vi "Gage_Core.vi"(8 "error in":errorcluster, 9 "SignalBufferQueue in":refnum<queue>, 10 "DWFCtrlQueue in":refnum<queue>) -> (0 "error out":errorcluster)   [LabVIEW 2013, in "Gage.lvlib"]
uses:
  <instrlib>/GageLv_uic/Gage.lvlib
  <instrlib>/AnalogDiscSDKLv/VIs/DWF_CtrlQueue.ctl
  <instrlib>/AnalogDiscSDKLv/VIs/DWF_State.ctl
  <instrlib>/GageLv_uic/VI/Gage_Configs.ctl
  <instrlib>/GageLv_uic/VI/Gage_PrivateStats.ctl
  <instrlib>/GageLv_uic/VI/Gage_DAQStatus.ctl
  <instrlib>/AnalogDiscSDKLv/VIs/DWF_Signal.ctl
  <vilib>/Utility/error.llb/DialogType.ctl
  <instrlib>/GageLv_uic/VI/SetSecondaryDataVIRef_Typedef.ctl
  <vilib>/Utility/error.llb/Error Cluster From Error Code.vi
  <vilib>/ErrorRing/Error Ring.xnode
  <instrlib>/AnalogDiscSDKLv/AnalogDiscSDKLv.lvlib
  <userlib>/Utility/ErrorLog_lib.lvlib
panel:
  in  "StartAll":bool
  out "Core#":i32
  in  "Get_ConfigAll":bool
  out "LiveStat":T1
  in  "Gage_Config":T3={"Acquisition"={"Sample Rate"=100000000.0, "Mode"=0, "Start (0)"=8192.0, "Depth"=8192.0, "Segment Size"=100.0, "Trigger Delay"=0.0, "Trigger Timeout"=0.0, "Trigger Holdoff"=0.0, "Clock mode"=enum."Internal"}, "Channels"=[{"Coupling"=0, "Differential Input"=FALSE, "Direct-to-ADC"=FALSE, "Range"=2000, "Impedance"=50, "DC Offset"=0, "Filter"=0}], "Trigger"={"Slope"=0, "Level"=0, "Source"=0, "External Range"=2000, "External Coupling"=0, "External"=TRUE, "Disable"=FALSE, "External Impedance"=0}, "Mode(Gage)"=enum."Continuous"} {"Trigger"."External Impedance" items=["50 Ohm", "HiZ"]; "Trigger"."External Coupling" items=["DC", "AC"]; "Trigger"."External Range" min=2000 max=10000 step=8000; "Trigger"."Slope" items=["Rising", "Falling"]; "Trigger"."Level" min=-100 max=100; "Trigger"."Source" min=0 max=64 step=1; "Channels"."Impedance" min=50 max=1000000 step=999950; "Channels"."Coupling" items=["DC", "AC"]; "Acquisition"."Segment Size" min=256.0 step=128.0; "Acquisition"."Trigger Delay" min=0.0 step=128.0; "Acquisition"."Trigger Timeout" format="%.0p"; "Acquisition"."Trigger Holdoff" min=0.0 step=128.0; "Acquisition"."Depth" min=256.0 step=128.0; "Acquisition"."Mode" items=["Single", "Dual", "Quad", "Octal"]; "Acquisition"."Sample Rate" format="%.0p"}
  out "Graph":sgl[][](graph)
  in  "fConfig":bool
  in  "Reset":bool
  in  "CloseAll":bool
  in  "Close":bool
  in  "Enumerate":bool
  in  "Open":bool
  in  "Quit":bool
  in  "Start":bool
  in  "ConfigAll":bool
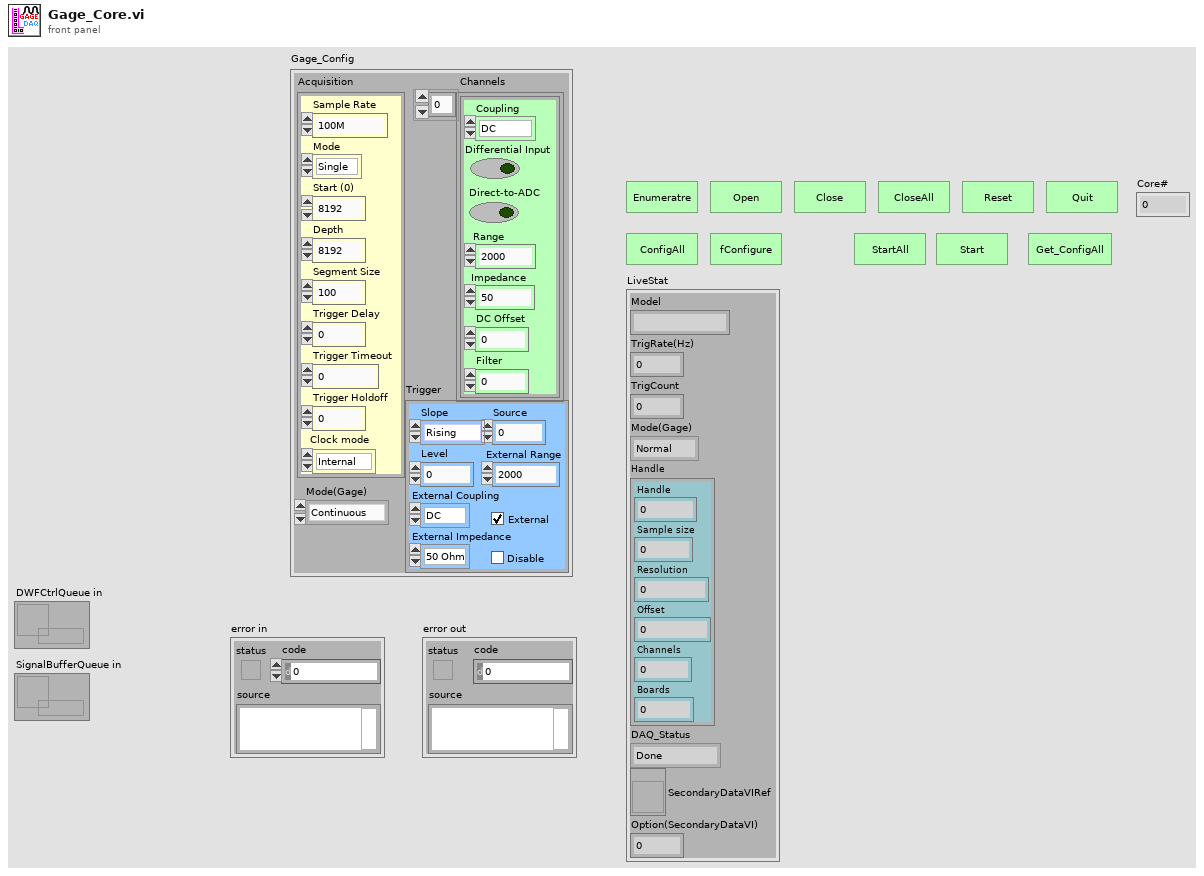
[diagram p1: front panel]
types:
  T1 = typedef "Gage.lvlib/Gage_PrivateStats.ctl" = cluster{"Model":string, "TrigRate(Hz)":dbl, "TrigCount":i32, "Mode(Gage)":enum16{"Normal", "Continuous", "MultiRecord", "HwAverage"}, "Handle":cluster{"Handle":u32, "Sample size":u32, "Resolution":i32, "Offset":i32, "Channels":u32, "Boards":u32}, "DAQ_Status":T2, "SecondaryDataVIRef":refnum<vi>, "Option(SecondaryDataVI)":i32}
  T2 = typedef "Gage.lvlib/Gage_DAQStatus.ctl" = enum16{"Done", "Armed", "Triggered", "Transfering"}
  T3 = typedef "Gage.lvlib/Gage_Configs.ctl" = cluster{"Acquisition":cluster{"Sample Rate":dbl, "Mode":u16, "Start (0)":dbl, "Depth":dbl, "Segment Size":dbl, "Trigger Delay":dbl, "Trigger Timeout":dbl, "Trigger Holdoff":dbl, "Clock mode":enum16{"Internal", "External", "Reference"}}, "Channels":cluster{"Coupling":u16, "Differential Input":bool, "Direct-to-ADC":bool, "Range":u32, "Impedance":u32, "DC Offset":i32, "Filter":i32}[], "Trigger":cluster{"Slope":u16, "Level":i32, "Source":i32, "External Range":u32, "External Coupling":u16, "External":bool, "Disable":bool, "External Impedance":u16}, "Mode(Gage)":enum16{"Normal", "Continuous", "MultiRecord", "HwAverage"}}
  T4 = typedef "DialogType.ctl" = u16
  T5 = typedef "AnalogDiscSDKLv.lvlib/DWF_Signal.ctl" = cluster{"tickcount":u32, "Signal":sgl[][], "SecondaryData":dbl[]}
  T6 = enum16{"Normal", "Continuous", "MultiRecord", "HwAverage"}
  T7 = typedef "AnalogDiscSDKLv.lvlib/DWF_CtrlQueue.ctl" = cluster{"DWF States":T8, "Variant":variant}
  T8 = typedef "AnalogDiscSDKLv.lvlib/DWF_State.ctl" = enum16{"Enumerate", "Open", "Close", "CloseAll", "Reset", "Quit", "==Settings==", "SetAcquisition_", "SetChannels_", "SetTrigger_", "SetAnalogTrigDetector_", "SetAll_AcquChTrig_", "fConfigurate", "fStart", "GetStatus", "_WaitForDone/Idle", "_GetData", "GetAcquisition", "GetChannels", "GetTrigger", "GetAll_AcquChTrig", "==Messaging==", "_PushDataOut", "GetStat_", "GetConfig_", "==ModeSetup==", "SetSignalBuffer_", "SetMode_", "SetSecondaryDataRef._", "==AnalogOut==", "GetChannelCount_AO", "fStart_AO", "SetChEnable_AO", "SetConfig_AO", "SetFuncData_AO", "SetOffset_AO_", "SetMasterNode_AO", "SetStates_AO", "SetSymetry_AO", "SetTriggerSource_AO", "==Trigger==", "ManualTrigger"}
  T9 = typedef "SetSecondaryDataVIRef_Typedef.ctl" = cluster{"SecondaryDataVIRef.":refnum<vi>, "Option":i32}
  T10 = cluster{"Handle":u32, "Sample size":u32, "Resolution":i32, "Offset":i32, "Channels":u32, "Boards":u32}
  T11 = cluster{"Sample Rate":dbl, "Mode":u16, "Start (0)":dbl, "Depth":dbl, "Segment Size":dbl, "Trigger Delay":dbl, "Trigger Timeout":dbl, "Trigger Holdoff":dbl, "Clock mode":enum16{"Internal", "External", "Reference"}}
  T12 = cluster{"Sample Rate":dbl, "Clock mode":enum16{"Internal", "External", "Reference"}, string, "Depth":dbl, "Segment Size":dbl, "Trigger Timeout":dbl, "Trigger Holdoff":dbl, "Trigger Delay":dbl}
  T13 = cluster{"Coupling":u16, "Differential Input":bool, "Direct-to-ADC":bool, "Range":u32, "Impedance":u32, "DC Offset":i32, "Filter":i32}[]
  T14 = cluster{string, "Differential Input":bool, "Direct-to-ADC":bool, "Range":u32, "Impedance":u32, "DC Offset":i32, "Filter":i32}
  T15 = cluster{"Slope":u16, "Level":i32, "Source":i32, "External Range":u32, "External Coupling":u16, "External":bool, "Disable":bool, "External Impedance":u16}
  T16 = cluster{string, "Level":i32, "Source":i32, "External Range":u32, string, "External":bool, "Disable":bool, string}
  T17 = cluster{string, "Level":i32, "Source":i32, "External Range":u32, string, "External":bool, "Disable":bool, string}[]
  T18 = cluster{"Handle":u32, "Sample Size":u32, "Resolution":i32, "Offset":i32, "Channels":u32, "Boards":u32}
  T19 = cluster{"Coupling":u16, "Differential Input":bool, "Direct-to-ADC":bool, "Range":u32, "Impedance":u32, "DC Offset":i32, "Filter":i32}
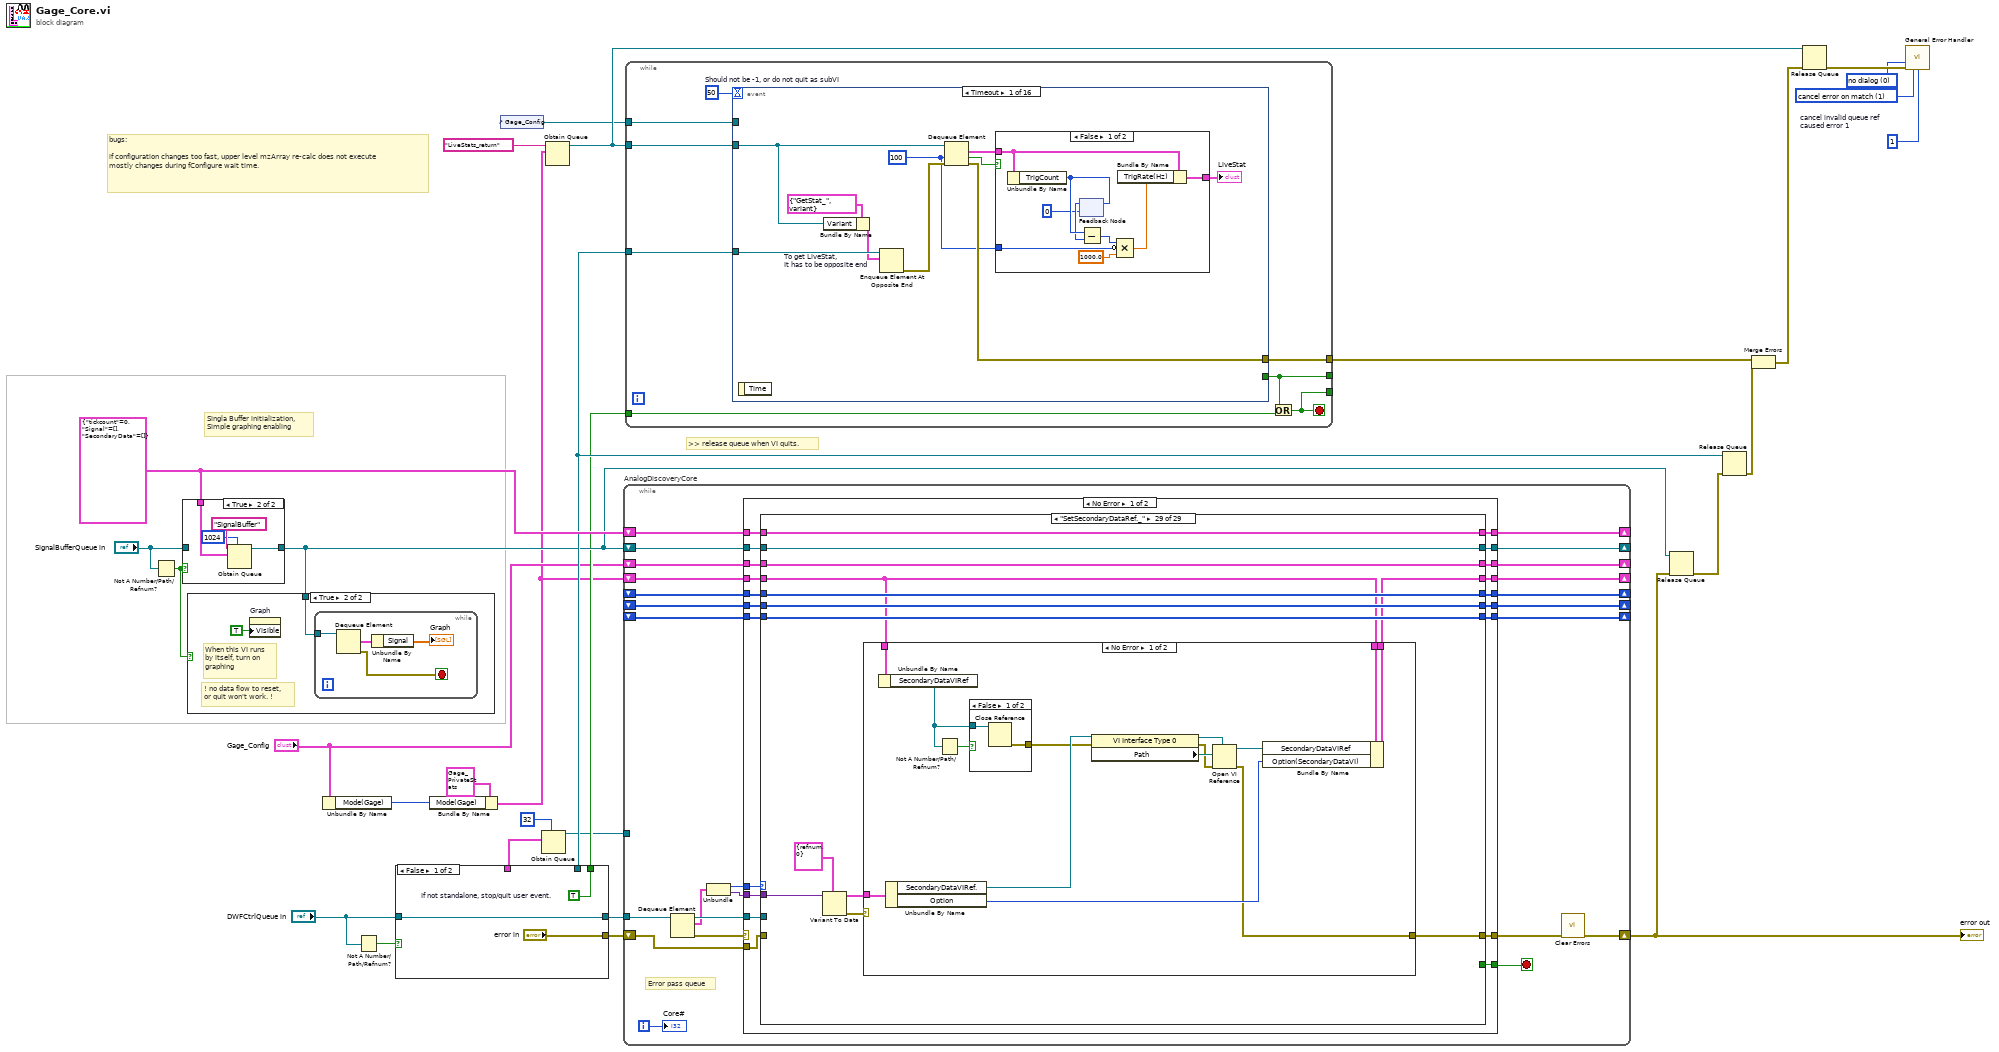
[diagram p0: block diagram]
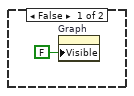
[diagram p2: hidden frame]
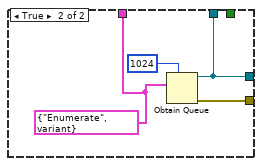
[diagram p4: hidden frame]
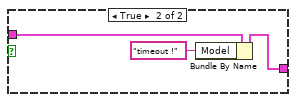
[diagram p5: hidden frame]
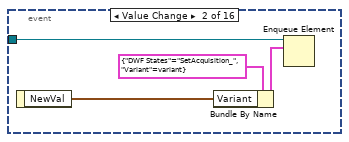
[diagram p6: hidden frame]
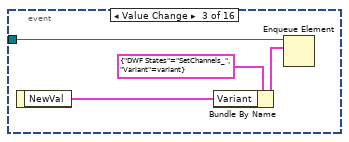
[diagram p7: hidden frame]
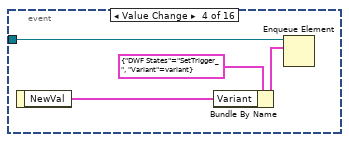
[diagram p8: hidden frame]
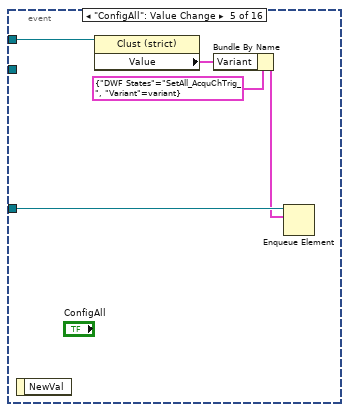
[diagram p9: hidden frame]
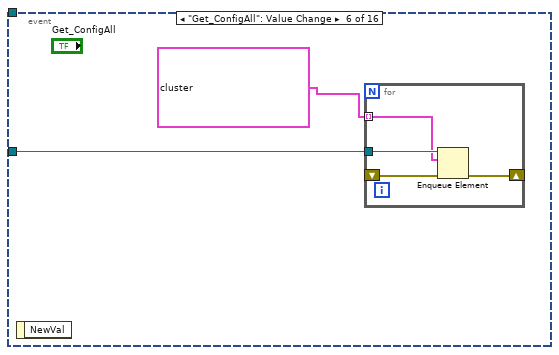
[diagram p10: hidden frame]
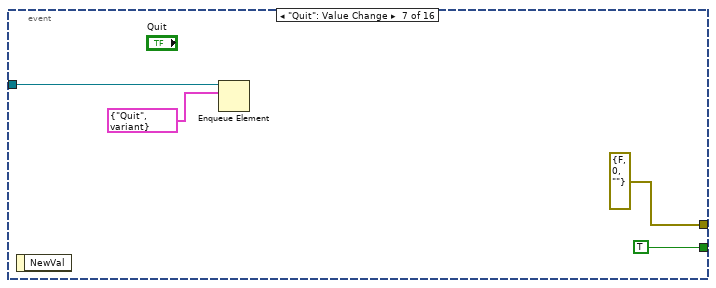
[diagram p11: hidden frame]
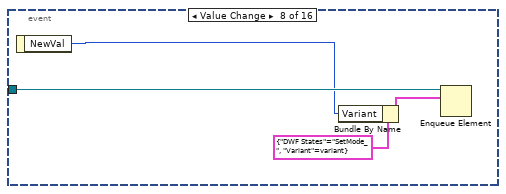
[diagram p12: hidden frame]
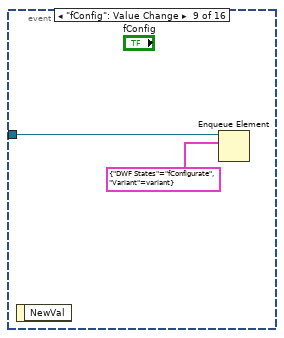
[diagram p13: hidden frame]
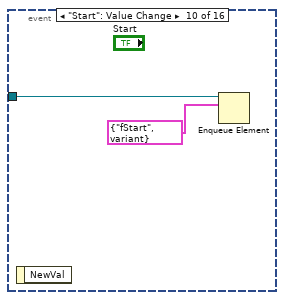
[diagram p14: hidden frame]
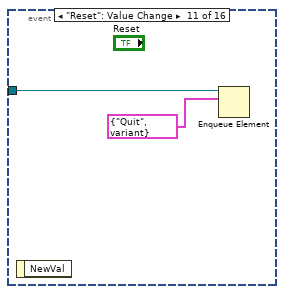
[diagram p15: hidden frame]
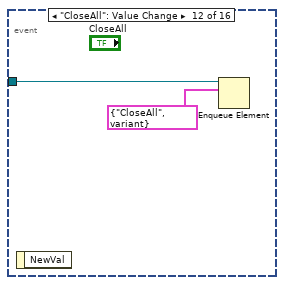
[diagram p16: hidden frame]
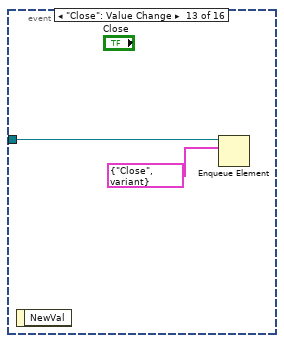
[diagram p17: hidden frame]
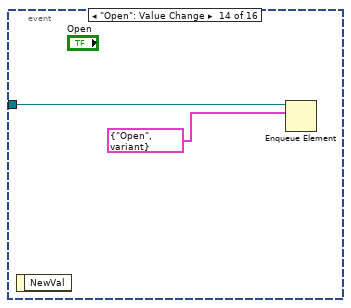
[diagram p18: hidden frame]
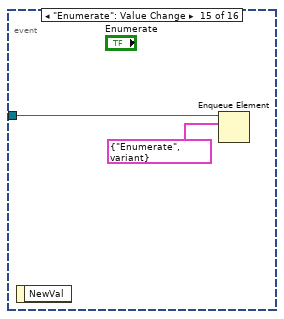
[diagram p19: hidden frame]
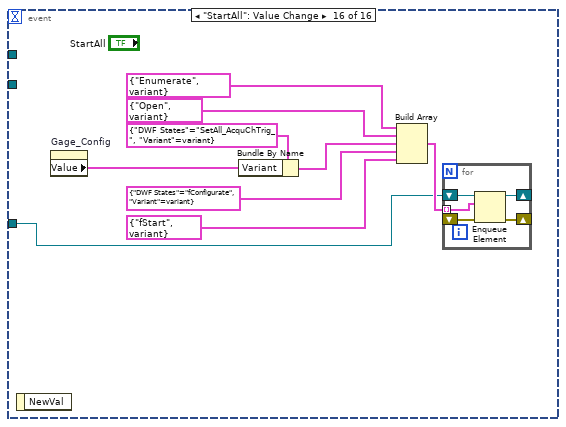
[diagram p20: hidden frame]
diagram:
  w11 = 1  # cancel invalid queue ref caused error 1
  w12 = 1 items=["no exception", "cancel error on match", "set error on match"] ("[exception action] (none:0)")
  w13 = T4 0 items=["no dialog", "OK message", "continue or stop message", "OK message + warnings", "continue/stop + warnings"] ("type of dialog (OK msg:1)")
  w29 = T5 {"tickcount"=0, "Signal"=[], "SecondaryData"=[]} ("Signal_Typedef")
  # "bugs:\n\nif configuration changes too fast, upper level mzArray re-calc does not execute\nmostly changes during fConfigure wait time."
  # "Singla Buffer initialization,\nSimple graphing enabling"
  # ">> release queue when VI quits."
  n1 = Not A Number/Path/Refnum?(number/path/refnum="SignalBufferQueue in") -> (NaN/Path/Refnum?=w16:bool)
  n2 = case shown="True" w16 {
    tunnel: w29 -> [_ w34]
    tunnel: [w30 w33] -> w17
    tunnel: "SignalBufferQueue in" -> [w30 _]
    frame False {
    }
    frame True {
      n3 = Obtain Queue(max queue size (-1, unlimited)=1024, name (unnamed)="SignalBuffer", element data type=w34) -> (queue out=w33:refnum<queue>)  [unwired: 2 in, 2 out]
    }
  }
  n4 = case shown="True" w16 {
    tunnel: w17 -> [_ w37]
    frame False {
      n5 = property on="Graph" class="WFGraph (strict)"("Visible"=FALSE) -> ()  [unwired: 2 in, 2 out]
    }
    frame True {
      # "! no data flow to reset,\nor quit won't work. !"
      # "When this VI runs\nby itself, turn on \ngraphing"
      n6 = property on="Graph" class="WFGraph (strict)"("Visible"=TRUE) -> ()  [unwired: 2 in, 2 out]
      n7 = while {
        tunnel: w37 -> [w41]
        stop <- w38 stop-if-true
        n8 = Dequeue Element(queue=w41) -> (element=w40:T5, error out=w38:errorcluster)  [unwired: 2 in, 2 out]
        n9 = Unbundle By Name(w40) -> ("Signal"=→"Graph":sgl[][])
      }
    }
  }
  n10 = Unbundle By Name("Gage_Config") -> ("Mode(Gage)"=w7:T6)
  n11 = Not A Number/Path/Refnum?(number/path/refnum="DWFCtrlQueue in") -> (NaN/Path/Refnum?=w26:bool)
  n12 = case shown="False" w26 {
    tunnel: [w44 w46] -> w28
    tunnel: ["error in" w48] -> w27
    tunnel: "DWFCtrlQueue in" -> [w44 _]
    tunnel: [_ w46] -> w22
    tunnel: [w42 _] -> w10
    tunnel: [_ w45] -> w3
    frame False {
      w42 = TRUE  # If not standalone, stop/quit user event.
    }
    frame True {
      w45 = T7 {"DWF States"=enum."Enumerate", "Variant"=variant}
      n13 = Obtain Queue(max queue size (-1, unlimited)=1024, element data type=w45) -> (queue out=w46:refnum<queue>, error out=w48:errorcluster)  [unwired: 3 in, 1 out]
    }
  }
  n14 = Bundle By Name(cluster=T1 {"Model"="", "TrigRate(Hz)"=0.0, "TrigCount"=0, "Mode(Gage)"=enum."Normal", "Handle"={"Handle"=0, "Sample size"=0, "Resolution"=0, "Offset"=0, "Channels"=0, "Boards"=0}, "DAQ_Status"=enum."Done", "SecondaryDataVIRef"=refnum, "Option(SecondaryDataVI)"=0} ("PrivateStats(Live)"), "Mode(Gage)"=w7) -> (w4:T1)
  n15 = control-ref of="Gage_Config"() -> (w5:refnum<vi>)
  n16 = Obtain Queue(max queue size (-1, unlimited)=32, element data type=w3) -> (queue out=w2:refnum<queue>)  [unwired: 3 in, 2 out]
  n17 = Obtain Queue(name (unnamed)="LiveStats_return", element data type=w4) -> (queue out=w20:refnum<queue>)  [unwired: 3 in, 2 out]
  n18 = while "AnalogDiscoveryCore" {
    shift-right: [w72] -> _
    shift-left: w17 -> [w73]
    tunnel: w28 -> [w59]
    shift-right: [w49] -> w15
    shift-left: w27 -> [w61]
    shift-right: [w70] -> _
    shift-left: "Gage_Config" -> [w69]
    shift-right: [w53] -> _
    shift-left: w4 -> [w68]
    shift-right: [w62] -> _
    shift-left: _ -> [w66]
    shift-right: [w63] -> _
    shift-left: w29 -> [w67]
    shift-right: [w56] -> _
    shift-left: _ -> [w54]
    shift-right: [w57] -> _
    shift-left: _ -> [w55]
    tunnel: w2 -> [_]
    i -> [w51]
    stop <- w71 stop-if-true
    # "Error pass queue"
    n19 = Dequeue Element(queue=w59) -> (queue out=w58:refnum<queue>, element=w52:T7, error out=w60:errorcluster)  [unwired: 2 in, 1 out]
    n20 = Unbundle(w52) -> ("DWF States"=w65:T8, "Variant"=w64:variant)
    n21 = case shown="No Error" w60 {
      tunnel: w73 -> [w93 w907]
      tunnel: [w92 w907] -> w72
      tunnel: [w91 TRUE] -> w71
      tunnel: [w90 w905] -> w50
      tunnel: [w89 w908] -> w70
      tunnel: w69 -> [w88 w908]
      tunnel: w68 -> [w87 w909]
      tunnel: w67 -> [w86 w906]
      tunnel: w66 -> [w85 w910]
      tunnel: w58 -> [w84 _]
      tunnel: w65 -> [w83 _]
      tunnel: w64 -> [w82 _]
      tunnel: [w81 w906] -> w63
      tunnel: [w80 w910] -> w62
      tunnel: [w79 w909] -> w53
      tunnel: w61 -> [w78 _]
      tunnel: [w77 w904] -> w57
      tunnel: [w76 w903] -> w56
      tunnel: w55 -> [w75 w904]
      tunnel: w54 -> [w74 w903]
      frame No Error {
        n22 = case shown="\"SetSecondaryDataRef._\"" w83 {
          tunnel: w93 -> [w101 w110 w138 w151 w167 w182 w199 w217 w239 w297 w341 w386 w435 w480 w511 w533 w584 w634 w649 w692 w703 w715 w740 w802 w815 w828 w841 w866 w879]
          tunnel: [w101 w110 w138 w151 w167 w182 w199 w217 w239 w297 w341 w386 w435 w480 w511 w533 w584 w634 w649 w692 w703 w715 w740 w802 w815 w828 w842 w866 w879] -> w92
          tunnel: [_ _ _ _ _ _ w193 _ _ _ _ _ _ _ _ _ _ _ _ _ _ _ _ _ _ _ _ _ _] -> w91
          tunnel: w84 -> [_ _ _ _ _ w178 w190 _ _ _ _ w383 w418 w474 _ w535 w579 _ _ _ w696 _ w736 _ _ _ _ _ _]
          tunnel: w78 -> [w100 w106 w134 w145 w166 w177 w191 _ w231 w288 w332 w377 w419 w465 w507 w534 w577 w633 w648 w691 w695 _ w738 w796 w806 _ w838 w855 _]
          tunnel: [w100 w106 errorcluster {"status"=FALSE, "code"=0, "source"=""} ("error out") w140 w159 w176 w192 w212 w227 w289 w333 w382 w415 w468 w507 w528 w581 w611 w637 w666 w694 w710 w737 w795 w807 w823 w839 w856 w867] -> w90
          tunnel: [w99 w109 w137 w150 w165 w181 w198 w216 w236 w294 w338 w380 w434 w479 w510 w532 w587 w628 w644 w684 w699 w714 w729 w794 w808 w827 w847 w865 w878] -> w89
          tunnel: w88 -> [w99 w109 w137 w150 w165 w181 w198 w216 w234 w292 w336 w380 w434 w479 w510 w532 w587 w630 w642 w690 w699 w714 w729 w794 w808 w827 w847 w865 w878]
          tunnel: [w98 w108 w129 w147 w160 w175 w195 w215 w237 w295 w339 w374 w432 w477 w506 w525 w575 w624 w643 w685 w702 w713 w735 w791 w814 w826 w846 w862 w873] -> w79
          tunnel: w87 -> [w98 w108 w135 w148 w160 w175 w195 w215 w237 w295 w339 w374 w432 w477 w502 w526 w573 w629 w643 w685 w702 w713 w735 w791 w814 w826 w846 w861 w868]
          tunnel: w86 -> [w97 w107 w136 w149 w164 w180 w197 w214 w238 w296 w340 w385 w433 w478 w509 w531 w583 w632 w647 w689 w701 w712 w733 w801 w813 w825 w845 w864 w877]
          tunnel: w85 -> [w96 w105 _ w146 w163 w179 w196 w213 w228 w286 w330 w384 w431 w473 w508 w527 w586 w631 w646 w688 w700 w711 w727 w800 w812 w824 w844 w863 w876]
          tunnel: w82 -> [_ _ w133 _ _ _ _ _ w235 w293 w337 w381 _ _ _ _ _ _ _ _ _ _ _ w797 w811 _ w843 w860 w871]
          tunnel: [w97 w107 w136 w149 w164 w180 w197 w214 w238 w296 w340 w385 w433 w478 w509 w531 w582 w632 w647 w689 w701 w712 w733 w801 w813 w825 w845 w864 w877] -> w81
          tunnel: [w96 w105 w119 w146 w163 w179 w196 w213 w229 w286 w330 w384 w431 w473 w508 w527 w576 w631 w646 w688 w700 w711 w726 w800 w812 w824 w844 w863 w876] -> w80
          tunnel: [w95 w103 w118 w144 w162 w169 w189 w211 w226 w285 w329 w376 w429 w472 w505 w515 w567 w618 w639 w687 w698 w709 w724 w793 w805 w822 w835 w854 w875] -> w77
          tunnel: [w94 w102 w117 w143 w161 w168 w188 w210 w225 w284 w328 w375 w428 w471 w504 w514 w566 w617 w638 w686 w697 w708 w722 w792 w804 w821 w834 w853 w874] -> w76
          tunnel: w75 -> [w95 w103 _ w144 w162 w169 w189 w211 w224 w285 w329 w376 w429 w472 w505 w515 w570 w618 w639 w687 w698 w709 w725 w793 w805 w822 w835 w854 w875]
          tunnel: w74 -> [w94 w102 _ w143 w161 w168 w188 w210 w223 w284 w328 w375 w428 w471 w504 w514 w569 w617 w638 w686 w697 w708 w723 w792 w804 w821 w834 w853 w874]
          frame Default {
          }
          frame "Enumerate" {
            n23 = call <instrlib>:"CsTool-Initialize.vi"() -> ("Number Of Systems"=w104:i32)  [unwired: 1 out]
            n24 = call <instrlib>:"CsTool-ErrorHandler.vi"("Error Code"=w104) -> ()  [unwired: 2 in, 1 out]
          }
          frame "Open" {
            w115 = 128000 ("dimension size")
            w116 = 2 ("16KSa, per spec")
            n25 = Variant To Data(error in=w134, type="", Variant=w133) -> (data=w128:string, error out=w131:errorcluster)
            n26 = Select(t="any", s=TRUE, f=w128) -> (s? t:f=w127:string)
            n27 = call <instrlib>:"CsTool-GetSystem.vi"("Board Name (Any)"=w127) -> ("Error Code"=w130:i32, "Handle Cluster"=w113:T10)  [unwired: 3 in]
            n28 = call <instrlib>:"CsTool-GetSystemName.vi"("Handle Cluster"=w113) -> ()  [unwired: 2 out]
            n29 = call <instrlib>:"CsTool-ErrorHandler.vi"("Error Code"=w130, "Handle Cluster"=w113) -> ("Error String"=w114:string)  [unwired: 1 in]
            n30 = call <instrlib>:"CsTool-GetSystemInfo.vi"("Handle Cluster"=w113) -> ()  [unwired: 7 out]
            n31 = Bundle By Name(cluster=w135, "Handle"=w113, "Model"=w127, "TrigRate(Hz)"=0.0, "TrigCount"=0) -> (w129:T1)
            n32 = Bundle By Name(cluster=w131, "source"=w114) -> ()  [unwired: 1 out]
            n33 = Wait (ms)(milliseconds to wait=u32 0) -> ()  [unwired: 1 out]
            n34 = Initialize Array(0 ("Numeric"), w116, w115) -> (w119:i32[][])
            n35 = Initialize Array(i16 0 ("Numeric"), w116, w115) -> (w118:i16[][])
            n36 = Initialize Array(u8 0 ("Numeric"), w116, w115) -> (w117:u8[][])
          }
          frame "Close" {
            n37 = Unbundle By Name(w148) -> ("Handle"=w141:T10)
            n38 = call <instrlib>:"CsTool-AbortCapture.vi"("Handle Cluster"=w141) -> ("Error Code"=w142:i32)
            n39 = call <instrlib>:"CsTool-ErrorHandler.vi"("Error Code"=w142, "Handle Cluster"=w141) -> ("Error String"=w139:string)  [unwired: 1 in]
            n40 = disable-structure shown="Enabled" {
              disable-tunnel: w148 -> [w154 w155]
              disable-tunnel: [w153 w155] -> w147
              frame Enabled {
                n41 = Bundle By Name(cluster=w154, "Handle.Handle"=u32 0) -> (w153:T1)
              }
              frame Disabled {
              }
            }
            n42 = Bundle By Name(cluster=w145, "source"=w139) -> (w140:errorcluster)
          }
          frame "CloseAll" {
            # "not really useful here."
            n43 = Unbundle By Name(w160) -> ("Handle"=w158:T10)
            n44 = call <instrlib>:"CsTool-AbortCapture.vi"("Handle Cluster"=w158) -> ("Error Code"=w157:i32)
            n45 = call <instrlib>:"CsTool-ErrorHandler.vi"("Error Code"=w157, "Handle Cluster"=w158) -> ("Error String"=w156:string)  [unwired: 1 in]
            n46 = Bundle By Name(cluster=w166, "source"=w156) -> (w159:errorcluster)
          }
          frame "Reset" {
            n47 = Unbundle By Name(w175) -> ("Model"=w173:string)
            n48 = Bundle By Name(cluster=T7 {"DWF States"=enum."Open", "Variant"=variant} ("element"), "Variant"=w173) -> (w172:T7)
            n49 = Build Array(w172, T7 {"DWF States"=enum."Close", "Variant"=variant} ("element")) -> (w170:T7[])
            n50 = for {
              tunnel: w178 -> [w186]
              tunnel: w170 -> [w183] mode=indexing
              shift-right: [w184] -> w176
              shift-left: w177 -> [w185]
              n51 = Enqueue Element At Opposite End(queue=w186, element=w183, error in (no error)=w185) -> (error out=w184:errorcluster)  [unwired: 1 in, 2 out]
            }
          }
          frame "Quit" {
            n52 = Unbundle By Name(w195) -> ("Handle"=w187:T10, "Handle.Handle"=w194:u32)
            n53 = case "Check handle leak??" shown="0" w194 {
              tunnel: [_ TRUE] -> w193
              tunnel: [w201 _] -> w192
              tunnel: w191 -> [w202 _]
              tunnel: w190 -> [w203 _]
              tunnel: w187 -> [_ w208]
              frame Default {
                n54 = for {
                  tunnel: w203 -> [w207]
                  tunnel: T7[] [{"DWF States"=enum."Quit", "Variant"=variant}, {"DWF States"=enum."Close", "Variant"=variant}] -> [w204] mode=indexing
                  shift-right: [w205] -> w201
                  shift-left: w202 -> [w206]
                  n55 = Enqueue Element At Opposite End(queue=w207, element=w204, error in (no error)=w206) -> (error out=w205:errorcluster)  [unwired: 1 in, 2 out]
                }
              }
              frame 0 {
                n56 = call <instrlib>:"CsTool-FreeSystem.vi"("Handle Cluster"=w208) -> ()  [unwired: 1 out]
              }
            }
          }
          frame "==Settings==" {
            # "Invalid frame"
            n57 = xnode "Error Ring"() -> ("error out"=w212:errorcluster)
          }
          frame "SetAcquisition_" {
            n58 = Unbundle By Name(w234) -> ("Acquisition"=w233:T11)
            n59 = Variant To Data(error in=w231, type=w233, Variant=w235) -> (data=w232:T11, error out=w230:errorcluster)
            n60 = Bundle By Name(cluster=w234, "Acquisition"=w232) -> (w236:T3)
            n61 = case shown="No Error" w230 {
              selector: w230 -> [w250 _]
              tunnel: w237 -> [w269 _]
              tunnel: w232 -> [w262 _]
              tunnel: [w254 w278] -> w229
              tunnel: w228 -> [_ w278]
              tunnel: [w249 w277] -> w227
              tunnel: [w253 w276] -> w226
              tunnel: [w252 w275] -> w225
              tunnel: w224 -> [_ w276]
              tunnel: w223 -> [_ w275]
              frame No Error {
                n62 = Unbundle By Name(w262) -> ("Mode"=w244:u16, "Sample Rate"=w268:dbl, "Clock mode"=w267:enum16{"Internal", "External", "Reference"})
                n63 = Unbundle By Name(w262) -> ("Depth"=w258:dbl, "Segment Size"=w266:dbl, "Trigger Timeout"=w265:dbl, "Trigger Holdoff"=w264:dbl, "Trigger Delay"=w263:dbl)
                n64 = Unbundle By Name(w269) -> ("Handle"=w247:T10)
                n65 = Index Array(array=string[] ["Single", "Dual", "Quad", "Octal"], index=w244) -> (element=w259:string)
                n66 = Scale By Power Of 2(n=w244, x=ext 1.0) -> (x*2^n=w245:ext)
                n67 = To Long Integer(number=w245) -> (32bit integer=w242:i32)
                n68 = Bundle("Sample Rate"=w268, "Clock mode"=w267, w259, "Depth"=w258, "Segment Size"=w266, "Trigger Timeout"=w265, "Trigger Holdoff"=w264, "Trigger Delay"=w263) -> (w261:T12)  [unwired: 1 in]
                n69 = flat-sequence {
                  tunnel: w247 -> [w273]
                  tunnel: [w273] -> w246
                  frame #0 {
                    n70 = call <instrlib>:"CsTool-AbortCapture.vi"("Handle Cluster"=w273) -> ()  [unwired: 1 out]
                    n71 = Wait (ms)(milliseconds to wait=u32 0) -> ()  [unwired: 1 out]
                  }
                }
                n72 = To Long Integer(number=w258) -> (32bit integer=w257:i32)
                n73 = call <instrlib>:"CsTool-ConfigureAcquisition.vi"("Handle Cluster"=w246, "Acquisition"=w261) -> ("Error Code"=w240:i32)  [unwired: 3 in]
                n74 = In Range and Coerce(upper limit=512000, x=w257, lower limit=1) -> (coerced(x)=w251:i32)  [unwired: 1 out]
                n75 = call <instrlib>:"CsTool-ErrorHandler.vi"("Error Code"=w240, "Handle Cluster"=w246) -> ("Error String"=w248:string)  [unwired: 1 in]
                n76 = Less Than 0?(x=w240) -> (x < 0?=w241:bool)
                n77 = Bundle By Name(cluster=w250, "status"=w241, "source"=w248) -> (w249:errorcluster)
                n78 = Initialize Array(0 ("Numeric"), w242, w251) -> (w254:i32[][])
                n79 = Initialize Array(i16 0 ("Numeric"), w242, w251) -> (w253:i16[][])
                n80 = Initialize Array(u8 0 ("Numeric"), w242, w251) -> (w252:u8[][])
              }
              frame Error {
                n81 = xnode "Error Ring"() -> ("error out"=w277:errorcluster)
              }
            }
          }
          frame "SetChannels_" {
            n82 = Unbundle By Name(w292) -> ("Channels"=w291:T13)
            n83 = Variant To Data(error in=w288, type=w291, Variant=w293) -> (data=w290:T13, error out=w287:errorcluster)
            n84 = Bundle By Name(cluster=w292, "Channels"=w290) -> (w294:T3)
            n85 = case shown="No Error" w287 {
              selector: w287 -> [w304 _]
              tunnel: w295 -> [w307 _]
              tunnel: w290 -> [w306 _]
              tunnel: [w301 w322] -> w289
              frame No Error {
                n86 = for {
                  tunnel: w306 -> [w311] mode=indexing
                  shift-right: [w321] -> w305
                  shift-left: w304 -> [w321]
                  tunnel: [w310] -> w303 mode=indexing
                  n87 = Unbundle By Name(w311) -> ("Coupling"=w314:u16, "Differential Input"=w312:bool, "Direct-to-ADC"=w315:bool, "Range"=w316:u32, "Impedance"=w317:u32, "DC Offset"=w318:i32, "Filter"=w319:i32)
                  n88 = Index Array(array=string[] ["DC\n", "AC"] ("Strings []"), index=w314) -> (element=w313:string)
                  n89 = Bundle(w313, "Differential Input"=w312, "Direct-to-ADC"=w315, "Range"=w316, "Impedance"=w317, "DC Offset"=w318, "Filter"=w319) -> (w310:T14)  [unwired: 1 in]
                }
                n90 = Unbundle By Name(w307) -> ("Handle"=w299:T10)
                n91 = flat-sequence {
                  tunnel: w299 -> [w308]
                  tunnel: [w308] -> w298
                  frame #0 {
                    n92 = call <instrlib>:"CsTool-AbortCapture.vi"("Handle Cluster"=w308) -> ()  [unwired: 1 out]
                    n93 = Wait (ms)(milliseconds to wait=u32 0) -> ()  [unwired: 1 out]
                  }
                }
                n94 = call <instrlib>:"CsTool-ConfigureChannelArray.vi"("Channels"=w303, "Handle Cluster"=w298) -> ("Error Code"=w302:u32)
                n95 = call <instrlib>:"CsTool-ErrorHandler.vi"("Error Code"=w302, "Handle Cluster"=w298) -> ("Error String"=w300:string)  [unwired: 1 in]
                n96 = Bundle By Name(cluster=w305, "source"=w300) -> (w301:errorcluster)
              }
              frame Error {
                n97 = xnode "Error Ring"() -> ("error out"=w322:errorcluster)
              }
            }
          }
          frame "SetTrigger_" {
            n98 = Unbundle By Name(w336) -> ("Trigger"=w335:T15)
            n99 = Variant To Data(error in=w332, type=w335, Variant=w337) -> (data=w334:T15, error out=w331:errorcluster)
            n100 = Bundle By Name(cluster=w336, "Trigger"=w334) -> (w338:T3)
            n101 = case shown="No Error" w331 {
              selector: w331 -> [w364 _]
              tunnel: w339 -> [w365 _]
              tunnel: w334 -> [w356 _]
              tunnel: [w345 w368] -> w333
              frame No Error {
                n102 = Unbundle By Name(w356) -> ("Slope"=w352:u16, "Level"=w360:i32, "Source"=w359:i32, "External Range"=w358:u32, "External Coupling"=w351:u16, "External"=w363:bool, "Disable"=w362:bool, "External Impedance"=w350:u16)
                n103 = Unbundle By Name(w365) -> ("Handle"=w342:T10)
                n104 = Index Array(array=string[] ["Rising", "Falling"] ("Strings [] 3"), index=w352) -> (element=w349:string)
                n105 = Index Array(array=string[] ["DC", "AC"] ("Strings [] 2"), index=w351) -> (element=w348:string)
                n106 = Index Array(array=string[] ["50 Ohm", "HiZ"] ("Strings []"), index=w350) -> (element=w347:string)
                n107 = Bundle(w349, "Level"=w360, "Source"=w359, "External Range"=w358, w348, "External"=w363, "Disable"=w362, w347) -> (w361:T16)  [unwired: 1 in]
                n108 = Build Array(w361) -> (w357:T17)
                n109 = flat-sequence {
                  tunnel: w342 -> [w366]
                  tunnel: [w366] -> w343
                  frame #0 {
                    n110 = call <instrlib>:"CsTool-AbortCapture.vi"("Handle Cluster"=w366) -> ()  [unwired: 1 out]
                    n111 = Wait (ms)(milliseconds to wait=u32 0) -> ()  [unwired: 1 out]
                  }
                }
                n112 = call <instrlib>:"CsTool-ConfigureTriggerArray.vi"("Triggers"=w357, "Handle Cluster"=w343) -> ("Error Code"=w346:i32)
                n113 = call <instrlib>:"CsTool-ErrorHandler.vi"("Error Code"=w346, "Handle Cluster"=w343) -> ("Error String"=w344:string)  [unwired: 1 in]
                n114 = Bundle By Name(cluster=w364, "source"=w344) -> (w345:errorcluster)
              }
              frame Error {
                n115 = xnode "Error Ring"() -> ("error out"=w368:errorcluster)
              }
            }
          }
          frame "SetAll_AcquChTrig_" {
            n116 = Variant To Data(type=w380, Variant=w381) -> (data=w378:T3, error out=w379:errorcluster)  [unwired: 1 in]
            n117 = case shown="No Error" w379 {
              tunnel: w383 -> [w404 _]
              tunnel: [w403 w409] -> w382
              tunnel: w378 -> [w402 _]
              tunnel: w377 -> [w401 _]
              frame No Error {
                n118 = Unbundle By Name(w402) -> ("Mode(Gage)"=w391:T6, "Acquisition"=w399:T11, "Channels"=w397:T13, "Trigger"=w395:T15)
                n119 = Bundle By Name(cluster=T7 {"DWF States"=enum."SetMode_", "Variant"=variant} ("element"), "Variant"=w391) -> (w388:T7)
                n120 = Bundle By Name(cluster=T7 {"DWF States"=enum."SetAcquisition_", "Variant"=variant} ("element"), "Variant"=w399) -> (w389:T7)
                n121 = Bundle By Name(cluster=T7 {"DWF States"=enum."SetChannels_", "Variant"=variant} ("element"), "Variant"=w397) -> (w387:T7)
                n122 = Bundle By Name(cluster=T7 {"DWF States"=enum."SetTrigger_", "Variant"=variant} ("element"), "Variant"=w395) -> (w394:T7)
                n123 = Build Array(w388, w389, w387, w394) -> (w393:T7[])
                n124 = Reverse 1D Array(array=w393) -> (reversed array=w390:T7[])
                n125 = for "Has to be at the \nopposite end, otherwise\nrace condition" {
                  tunnel: w404 -> [w408]
                  shift-right: [w407] -> w403
                  shift-left: w401 -> [w406]
                  tunnel: w390 -> [w405] mode=indexing
                  n126 = Enqueue Element At Opposite End(queue=w408, element=w405, error in (no error)=w406) -> (error out=w407:errorcluster)  [unwired: 1 in, 2 out]
                }
              }
              frame Error {
                n127 = xnode "Error Ring"() -> ("error out"=w409:errorcluster)
              }
            }
          }
          frame "fConfigurate" {
            # "If dependancy of ErrorLog missing, \njust remove errorlog vi."
            # "fConfigurate => Commit (as in Gage SDK)"
            n128 = Unbundle By Name(w432) -> ("Handle"=w430:T10)
            n129 = Flush Queue(queue=w418, error in (no error)=w419) -> (queue out=w424:refnum<queue>, remaining elements=w422:T7[], error out=w423:errorcluster)
            n130 = for "Remove unfinished acquisition process" {
              shift-right: [w442] -> _
              shift-left: w424 -> [w443]
              shift-right: [w440] -> w420
              shift-left: w423 -> [w441]
              tunnel: w422 -> [w436] mode=indexing
              tunnel: T7[] [{"DWF States"=enum."_WaitForDone/Idle", "Variant"=variant}, {"DWF States"=enum."_GetData", "Variant"=variant}, {"DWF States"=enum."_PushDataOut", "Variant"=variant}] ("remaining elements") -> [w439]
              n131 = Search 1D Array(1D array=w439, element=w436) -> (index of element=w438:i32)  [unwired: 1 in]
              n132 = Greater Or Equal To 0?(x=w438) -> (x >= 0?=w437:bool)
              n133 = case shown="False" w437 {
                tunnel: w443 -> [w448 w450]
                tunnel: [w447 w450] -> w442
                tunnel: w441 -> [w446 w449]
                tunnel: [w445 w449] -> w440
                tunnel: w436 -> [w444 _]
                frame False {
                  n134 = Enqueue Element(queue=w448, element=w444, error in (no error)=w446) -> (queue out=w447:refnum<queue>, error out=w445:errorcluster)  [unwired: 1 in, 1 out]
                }
                frame True {
                }
              }
            }
            n135 = flat-sequence {
              tunnel: w430 -> [w451]
              tunnel: [w451] -> w427
              tunnel: w427 -> [w454]
              tunnel: [w455] -> w425
              tunnel: [w453] -> w416
              frame #0 {
                n136 = disable-structure shown="Enabled" {
                  disable-tunnel: w451 -> [w452 _]
                  frame Disabled {
                    n137 = call <instrlib>:"CsTool-AbortCapture.vi"("Handle Cluster"=w452) -> ()  [unwired: 1 out]
                  }
                  frame Enabled {
                  }
                }
              }
              frame #1 {
                n138 = call <instrlib>:"CsTool-Commit.vi"("Handle Cluster"=w454) -> ("Error Code"=w453:i32)  [unwired: 2 in, 1 out]
                n139 = call <instrlib>:"CsTool-ErrorHandler.vi"("StopOnError (true)"=FALSE, "Error Code"=w453, "Handle Cluster"=w454) -> ("Error String"=w455:string)
                n140 = case shown="True" FALSE {
                  tunnel: w454 -> [_ w459]
                  tunnel: w453 -> [_ w458]
                  frame False {
                  }
                  frame True {
                    n141 = call <instrlib>:"DisplayCurrentConfiguration.vi"("error code  in"=w458, "Handle Cluster"=w459) -> ()  [unwired: 10 in]
                  }
                }
              }
            }
            n142 = Less Than 0?(x=w416) -> (x < 0?=w417:bool)
            n143 = Bundle By Name(cluster=w420, "status"=w417, "source"=w425) -> (w426:errorcluster)
            n144 = call <userlib>:"ErrorLog.vi"("error in (no error)"=w426) -> ("error out"=w415:errorcluster)  [unwired: 10 in]
          }
          frame "fStart" {
            # "Known issue:\n\nIf too manu fStart send here, virtual system crash.\nhas to restart Lv"
            # "Prevent program termination, \nwhen capture executed \nbefore previous one finished\n\nCould not find how to detect\na unfinished capture\n\nIn GetDate frame, capture actions is \nguarentted finished, no need to do so."
            n145 = Unbundle By Name(w477) -> ("Handle"=w470:T10)
            n146 = Flush Queue(queue=w474, error in (no error)=w465) -> (queue out=w466:refnum<queue>, remaining elements=w461:T7[], error out=w463:errorcluster)
            n147 = flat-sequence {
              tunnel: w470 -> [w497]
              tunnel: [w497] -> w469
              tunnel: w469 -> [w499]
              tunnel: [w498] -> w467
              frame #0 {
                n148 = Wait (ms) "Prevent termination if too many \nfStart sent in short time."(milliseconds to wait=u32 50) -> ()  [unwired: 1 out]
                n149 = call <instrlib>:"CsTool-AbortCapture.vi"("Handle Cluster"=w497) -> ()  [unwired: 1 out]
              }
              frame #1 {
                n150 = call <instrlib>:"CsTool-Capture.vi"("Handle Cluster"=w499) -> ("Error Code"=w500:i32)
                n151 = call <instrlib>:"CsTool-ErrorHandler.vi"("Error Code"=w500, "Handle Cluster"=w499) -> ("Error String"=w498:string)  [unwired: 1 in]
              }
            }
            n152 = for "Remove unfinished acquisition process" {
              shift-right: [w487] -> w464
              shift-left: w466 -> [w488]
              shift-right: [w485] -> w462
              shift-left: w463 -> [w486]
              tunnel: w461 -> [w481] mode=indexing
              tunnel: T7[] [{"DWF States"=enum."_WaitForDone/Idle", "Variant"=variant}, {"DWF States"=enum."_GetData", "Variant"=variant}, {"DWF States"=enum."_PushDataOut", "Variant"=variant}] ("remaining elements") -> [w484]
              n153 = Search 1D Array(1D array=w484, element=w481) -> (index of element=w483:i32)  [unwired: 1 in]
              n154 = Greater Or Equal To 0?(x=w483) -> (x >= 0?=w482:bool)
              n155 = case shown="False" w482 {
                tunnel: w488 -> [w493 w495]
                tunnel: [w492 w495] -> w487
                tunnel: w486 -> [w491 w494]
                tunnel: [w490 w494] -> w485
                tunnel: w481 -> [w489 _]
                frame False {
                  n156 = Enqueue Element(queue=w493, element=w489, error in (no error)=w491) -> (queue out=w492:refnum<queue>, error out=w490:errorcluster)  [unwired: 1 in, 1 out]
                }
                frame True {
                }
              }
            }
            n157 = Enqueue Element(queue=w464, element=T7 {"DWF States"=enum."_WaitForDone/Idle", "Variant"=variant}, error in (no error)=w462) -> (error out=w475:errorcluster)  [unwired: 1 in, 2 out]
            n158 = Bundle By Name(cluster=w475, "source"=w467) -> (w468:errorcluster)
          }
          frame "GetStatus" {
            n159 = Unbundle By Name(w502) -> ("Handle"=w503:T10)
            n160 = call <instrlib>:"CsTool-QueryStatus.vi"("Handle Cluster"=w503) -> ("Status"=w501:i32)
            n161 = Bundle By Name(cluster=w502, "DAQ_Status"=w501) -> (w506:T1)
          }
          frame "_WaitForDone/Idle" {
            w521 = T8[] [enum."Close", enum."CloseAll", enum."Reset", enum."Quit"] items=["Enumerate", "Open", "Close", "CloseAll", "Reset", "Quit", "==Settings==", "SetAcquisition_", "SetChannels_", "SetTrigger_", "SetAnalogTrigDetector_", "SetAll_AcquChTrig_", "fConfigurate", "fStart", "GetStatus", "_WaitForDone/Idle", "_GetData", "GetAcquisition", "GetChannels", "GetTrigger", "GetAll_AcquChTrig", "==Messaging==", "_PushDataOut", "GetStat_", "GetConfig_", "==ModeSetup==", "SetSignalBuffer_", "SetMode_", "SetSecondaryDataRef._", "==AnalogOut==", "GetChannelCount_AO", "fStart_AO", "SetChEnable_AO", "SetConfig_AO", "SetFuncData_AO", "SetOffset_AO_", "SetMasterNode_AO", "SetStates_AO", "SetSymetry_AO", "SetTriggerSource_AO", "==Trigger==", "ManualTrigger"]
            # "to be considered \n\nwhat if system not configed??\nwhat status is that?"
            # "0 dne\n1 armed\n2 triggered\n3 transfering"
            n162 = Unbundle By Name(w526) -> ("Handle"=w516:T10)
            n163 = call <instrlib>:"CsTool-QueryStatus.vi"("Handle Cluster"=w516) -> ("Status"=w513:i32)
            n164 = Bundle By Name(cluster=w526, "DAQ_Status"=w513) -> (w525:T1)
            n165 = Preview Queue Element(queue=w535, timeout in ms (-1)=0, error in (no error)=w534) -> (queue out=w530:refnum<queue>, element=w523:T7, timed out?=w522:bool, error out=w529:errorcluster)
            n166 = Unbundle(w523) -> ("DWF States"=w518:T8)  [unwired: 1 out]
            n167 = Search 1D Array(1D array=w521, element=w518) -> (index of element=w520:i32)  [unwired: 1 in]
            n168 = Greater Or Equal To 0?(x=w520) -> (x >= 0?=w519:bool)
            n169 = Compound Arithmetic op=AND(w519, invert w522) -> (w517:bool)
            n170 = case shown="False" w517 {
              tunnel: w530 -> [w539 _]
              tunnel: w529 -> [w538 w556]
              tunnel: [w537 w556] -> w528
              tunnel: w513 -> [w536 _]
              frame False {
                n171 = case shown="1" w536 {
                  tunnel: w539 -> [w540 w551 w555]
                  tunnel: w538 -> [w543 w550 w554]
                  tunnel: [w542 w549 w553] -> w537
                  frame 1 {
                    # "armed ??"
                    # "Typically, this is caused by config change\nduring acquisition. \nPush fConfig and fStart to continure  acuisition."
                    # "armed, not configed??"
                    n172 = for {
                      shift-right: [w546] -> w542
                      shift-left: w543 -> [w547]
                      tunnel: T7[] [{"DWF States"=enum."_WaitForDone/Idle", "Variant"=variant}] -> [w545] mode=indexing
                      tunnel: w540 -> [w544]
                      n173 = Enqueue Element(queue=w544, element=w545, error in (no error)=w547) -> (error out=w546:errorcluster)  [unwired: 1 in, 2 out]
                    }
                  }
                  frame 0 {
                    # "Done"
                    n174 = Enqueue Element(queue=w551, element=T7 {"DWF States"=enum."_GetData", "Variant"=variant}, error in (no error)=w550) -> (error out=w549:errorcluster)  [unwired: 1 in, 2 out]
                  }
                  frame 2, Default {
                    # "triggered"
                    # "triggered, others"
                    n175 = Enqueue Element(queue=w555, element=T7 {"DWF States"=enum."_WaitForDone/Idle", "Variant"=variant}, error in (no error)=w554) -> (error out=w553:errorcluster)  [unwired: 1 in, 2 out]
                  }
                }
              }
              frame True {
              }
            }
            n176 = Wait (ms)(milliseconds to wait=u32 0) -> ()  [unwired: 1 out]
          }
          frame "_GetData" {
            w565 = u32 0  # Mode (0)
            # "For performance purposes.\nminimize memory allocation while callig C functions"
            # "No multiple record mode now."
            # "If 0 channel enabled, then this will generate\n an empty array output in queue"
            n177 = Enqueue Element(queue=w579, element=T7 {"DWF States"=enum."_PushDataOut", "Variant"=variant}, error in (no error)=w577) -> (error out=w563:errorcluster)  [unwired: 1 in, 2 out]
            n178 = Unbundle By Name(w587) -> ("Channels"=w571:T13, "Acquisition.Depth"=w568:dbl, "Mode(Gage)"=w560:T6)
            n179 = Unbundle By Name(w573) -> ("TrigCount"=w572:i32, "SecondaryDataVIRef"=w557:refnum<vi>, "Handle"=w561:T10)
            n180 = Array Size(array=w571) -> (size(s)=w564:i32)
            n181 = disable-structure shown="Disabled" {
              frame Disabled {
                n182 = call <instrlib>:"CsTool-TransferTimeStamp.vi"() -> ()  [unwired: 3 in, 3 out]
              }
              frame Enabled {
              }
            }
            n183 = for {
              N: w564 -> [_]
              tunnel: w586 -> [w601] mode=indexing
              tunnel: [w600] -> w576 mode=indexing
              tunnel: w561 -> [w599]
              tunnel: w570 -> [w598] mode=indexing
              tunnel: w569 -> [w597] mode=indexing
              tunnel: w568 -> [w596]
              tunnel: [w595] -> w567 mode=indexing
              tunnel: [w592] -> w566 mode=indexing
              tunnel: w565 -> [w594]
              tunnel: w560 -> [w593]
              tunnel: [w592] -> _
              shift-right: [w591] -> w562
              shift-left: w563 -> [w591]
              i -> [w590]
              n184 = call <instrlib>:"GageTransfer-LowOverheadMod.vi"("Handle Cluster"=w599, "Start (0)"=w593, "Length (4096)"=w596, "Buffer in I32"=w601, "Buffer in I16"=w598, "Buffer in U8"=w597, "Channel (0)"=w590, "Mode (0)"=w594) -> ("Buffer Out I32"=w600:i32[], "Buffer Out I16"=w595:i16[], "Buffer Out U8"=w592:u8[])  [unwired: 2 in, 3 out]
            }
            n185 = Unbundle By Name(w573) -> ("Mode(Gage)"=w580:T6)
            n186 = Not A Number/Path/Refnum?(number/path/refnum=w557) -> (NaN/Path/Refnum?=w558:bool)
            n187 = case shown="\"Continuous\"" w580 {
              tunnel: w562 -> [w602 w607 w608 w609]
              tunnel: [w602 w605 w608 w609] -> w581
              tunnel: w561 -> [_ w603 _ _]
              frame "Normal", Default {
              }
              frame "Continuous" {
                n188 = call <instrlib>:"CsTool-Capture.vi"("Handle Cluster"=w603) -> ("Error Code"=w606:i32)
                n189 = call <instrlib>:"CsTool-ErrorHandler.vi"("Error Code"=w606, "Handle Cluster"=w603) -> ("Error String"=w604:string)  [unwired: 1 in]
                n190 = Bundle By Name(cluster=w607, "source"=w604) -> (w605:errorcluster)
              }
              frame "MultiRecord" {
              }
              frame "HwAverage" {
              }
            }
            n191 = case shown="False" w558 {
              tunnel: [w589 _] -> w559
              tunnel: w557 -> [w588 _]
              frame False {
                n192 = call-by-ref "?"(reference=w588) -> ("SecondaryData"=w589:dbl[])  [unwired: 12 in, 2 out]
              }
              frame True {
              }
            }
            n193 = Increment(x=w572) -> (x+1=w574:i32)
            n194 = Tick Count (ms)() -> (millisecond timer value=w585:u32)
            n195 = Bundle By Name(cluster=w573, "TrigCount"=w574) -> (w575:T1)
            n196 = Bundle By Name(cluster=w583, "tickcount"=w585, "SecondaryData"=w559) -> (w582:T5)
          }
          frame "GetAcquisition" {
            # "Mode and Segment Count"
            n197 = Unbundle By Name(w629) -> ("Handle"=w613:T10)
            n198 = call <instrlib>:"CsTool-QueryAcquisitionParameters.vi"("Handle Cluster"=w613) -> ("Error Code"=w612:i32, "Trigger Holdoff"=w627:dbl, "Trigger Delay"=w626:dbl, "Output Handle Cluster"=w623:T18, "Sample Rate"=w625:dbl, "Clock Mode"=w622:enum16{"Internal", "External", "Reference"}, "Mode"=w615:string, "Trigger Timeout"=w619:dbl, "Segment Size"=w620:dbl, "Depth"=w621:dbl)  [unwired: 4 in, 1 out]
            n199 = call <instrlib>:"CsTool-ErrorHandler.vi"("Error Code"=w612, "Handle Cluster"=w613) -> ("Error String"=w610:string)  [unwired: 1 in]
            n200 = Bundle By Name(cluster=w633, "source"=w610) -> (w611:errorcluster)
            n201 = Bundle By Name(cluster=w629, "Handle"=w623) -> (w624:T1)
            n202 = Search 1D Array(1D array=string[] ["Single", "Dual", "Quad", "Octal"], element=w615) -> (index of element=w614:i32)  [unwired: 1 in]
            n203 = Bundle By Name(cluster=w630, "Acquisition.Sample Rate"=w625, "Acquisition.Mode"=w614, "Acquisition.Depth"=w621, "Acquisition.Segment Size"=w620, "Acquisition.Trigger Timeout"=w619, "Acquisition.Trigger Holdoff"=w627, "Acquisition.Trigger Delay"=w626, "Acquisition.Clock mode"=w622) -> (w628:T3)
          }
          frame "GetChannels" {
            n204 = Unbundle By Name(w643) -> ("Handle"=w645:T10)
            n205 = Unbundle By Name(w642) -> ("Channels"=w641:T13)
            n206 = for {
              tunnel: w645 -> [w651]
              tunnel: w641 -> [w663] mode=indexing
              tunnel: [w656] -> w640 mode=indexing
              tunnel: [w650] -> w636 mode=indexing
              i -> [w664]
              n207 = call <instrlib>:"CsTool-QueryChannelParameters.vi"("Handle Cluster"=w651, "Channel"=w664) -> ("Filter"=w657:u32, "Coupling"=w654:string, "Differential Input"=w662:bool, "Direct-to-ADC"=w658:bool, "Range (mV)"=w661:u32, "Impedance"=w660:u32, "DC Offset (mV)"=w659:u32, "Error Code"=w652:i32)
              n208 = call <instrlib>:"CsTool-ErrorHandler.vi"("Error Code"=w652, "Handle Cluster"=w651) -> ("Error String"=w650:string)  [unwired: 1 in]
              n209 = Search 1D Array(1D array=string[] ["DC", "AC"], element=w654) -> (index of element=w653:i32)  [unwired: 1 in]
              n210 = Bundle By Name(cluster=w663, "Differential Input"=w662, "Range"=w661, "Impedance"=w660, "DC Offset"=w659, "Direct-to-ADC"=w658, "Coupling"=w653, "Filter"=w657) -> (w656:T19)
            }
            n211 = Concatenate Strings(w636) -> (w635:string)
            n212 = Bundle By Name(cluster=w642, "Channels"=w640) -> (w644:T3)
            n213 = Bundle By Name(cluster=w648, "source"=w635) -> (w637:errorcluster)
          }
          frame "GetTrigger" {
            n214 = Unbundle By Name(w685) -> ("Handle"=w667:T10)
            n215 = call <instrlib>:"CsTool-QueryTriggerParameters.vi"("Handle Cluster"=w667, "Trigger"=u32 0) -> ("External Impedance"=w671:string, "External Range (mV)"=w683:u32, "External Coupling"=w674:string, "Error Code"=w668:i32, "Source"=w682:i32, "Slope"=w677:string, "Level"=w681:i32, "External Trigger"=w680:bool, "Disable Trigger"=w679:bool)  [unwired: 9 in]
            n216 = call <instrlib>:"CsTool-ErrorHandler.vi"("Error Code"=w668, "Handle Cluster"=w667) -> ("Error String"=w665:string)  [unwired: 1 in]
            n217 = Search 1D Array(1D array=string[] ["rising", "falling"], element=w677) -> (index of element=w676:i32)  [unwired: 1 in]
            n218 = Search 1D Array(1D array=string[] ["dc", "ac"], element=w674) -> (index of element=w673:i32)  [unwired: 1 in]
            n219 = Search 1D Array(1D array=string[] ["50 Ohm", "HiZ"], element=w671) -> (index of element=w670:i32)  [unwired: 1 in]
            n220 = Bundle By Name(cluster=w691, "source"=w665) -> (w666:errorcluster)
            n221 = Bundle By Name(cluster=w690, "Trigger.External Range"=w683, "Trigger.Source"=w682, "Trigger.Slope"=w676, "Trigger.Level"=w681, "Trigger.External"=w680, "Trigger.Disable"=w679, "Trigger.External Coupling"=w673, "Trigger.External Impedance"=w670) -> (w684:T3)
          }
          frame "GetAll_AcquChTrig" {
            n222 = for "Has to be at the \nopposite end, otherwise\nrace condition" {
              tunnel: w696 -> [w707]
              shift-right: [w706] -> w694
              shift-left: w695 -> [w705]
              tunnel: T7[] [{"DWF States"=enum."GetAcquisition", "Variant"=variant}, {"DWF States"=enum."GetChannels", "Variant"=variant}, {"DWF States"=enum."GetTrigger", "Variant"=variant}] -> [w704] mode=indexing
              n223 = Enqueue Element At Opposite End(queue=w707, element=w704, error in (no error)=w705) -> (error out=w706:errorcluster)  [unwired: 1 in, 2 out]
            }
          }
          frame "==Messaging==" {
            # "Invalid Frame"
            n224 = xnode "Error Ring"() -> ("error out"=w710:errorcluster)
          }
          frame "_PushDataOut" {
            # "In turbo mode, \nre-arming is done in \"_GetData\"\n\nNormal mode => no need to re-arming  daq"
            n225 = Unbundle By Name(w735) -> ("Mode(Gage)"=w739:T6)
            n226 = Unbundle By Name(w735) -> ("Handle.Resolution"=w721:i32, "Handle.Sample size"=w734:u32, "Handle.Offset"=w730:i32)
            n227 = Unbundle By Name(w729) -> ("Channels"=w728:T13)
            n228 = case shown="\"Continuous\", Default" w739 {
              tunnel: w738 -> [w785 w789]
              tunnel: [w785 w788] -> w737
              tunnel: w736 -> [_ w787]
              frame "Normal" {
              }
              frame "Continuous", Default {
                n229 = Enqueue Element(queue=w787, element=T7 {"DWF States"=enum."_WaitForDone/Idle", "Variant"=variant}, error in (no error)=w789) -> (error out=w788:errorcluster)  [unwired: 1 in, 2 out]
              }
            }
            n230 = case shown="2" w734 {
              tunnel: w723 -> [w744 w757 w773]
              tunnel: [w747 w762 w776] -> w731
              tunnel: w725 -> [w743 w758 w772]
              tunnel: w727 -> [w742 w759 w771]
              tunnel: w730 -> [w746 w761 w775]
              tunnel: w728 -> [w745 w760 w774]
              tunnel: [w742 w759 w771] -> w726
              tunnel: [w743 w758 w772] -> w724
              tunnel: [w744 w757 w773] -> w722
              tunnel: w721 -> [w741 w756 w770]
              frame 4 {
                n231 = for {
                  tunnel: w742 -> [w755] mode=indexing
                  tunnel: [w748] -> w747 mode=indexing
                  tunnel: w741 -> [w753]
                  tunnel: w746 -> [w752]
                  tunnel: w745 -> [w751] mode=indexing
                  n232 = Unbundle By Name(w751) -> ("DC Offset"=w750:i32, "Range"=w749:u32)
                  n233 = call <instrlib>:"ConvertTo_DBL.vi"("Input Range (mV)"=w749, "DC Offset (mV)"=w750, "Offset"=w752, "Resolution"=w753, "Interger Signal"=w755) -> ("Data (V)"=w754:sgl[])  [unwired: 6 in]
                  n234 = To Single Precision Float(number=w754) -> (single precision float=w748:sgl[])
                }
              }
              frame 2 {
                n235 = for {
                  tunnel: w758 -> [w769] mode=indexing
                  tunnel: [w763] -> w762 mode=indexing
                  tunnel: w756 -> [w768]
                  tunnel: w761 -> [w767]
                  tunnel: w760 -> [w766] mode=indexing
                  n236 = Unbundle By Name(w766) -> ("DC Offset"=w765:i32, "Range"=w764:u32)
                  n237 = call <instrlib>:"ConvertTo_DBL.vi"("Input Range (mV)"=w764, "DC Offset (mV)"=w765, "Offset"=w767, "Resolution"=w768, "Interger Signal"=w769) -> ("Data (V)"=w763:sgl[])  [unwired: 6 in]
                }
              }
              frame 1, Default {
                n238 = for {
                  tunnel: w773 -> [w784] mode=indexing
                  tunnel: [w777] -> w776 mode=indexing
                  tunnel: w770 -> [w782]
                  tunnel: w775 -> [w781]
                  tunnel: w774 -> [w780] mode=indexing
                  n239 = Unbundle By Name(w780) -> ("DC Offset"=w779:i32, "Range"=w778:u32)
                  n240 = call <instrlib>:"ConvertTo_DBL.vi"("Input Range (mV)"=w778, "DC Offset (mV)"=w779, "Offset"=w781, "Resolution"=w782, "Interger Signal"=w784) -> ("Data (V)"=w783:sgl[])  [unwired: 6 in]
                  n241 = To Single Precision Float(number=w783) -> (single precision float=w777:sgl[])
                }
              }
            }
            n242 = Bundle By Name(cluster=w733, "Signal"=w731) -> (w732:T5)
            n243 = Enqueue Element "Send/Push Data Out"(queue=w740, element=w732) -> ()  [unwired: 2 in, 3 out]
          }
          frame "GetStat_" {
            n244 = Variant To Data(error in=w796, type=refnum<queue> refnum ("queue out"), Variant=w797) -> (data=w799:refnum<queue>, error out=w798:errorcluster)
            n245 = Enqueue Element "Send Core Stat"(queue=w799, element=w791, error in (no error)=w798) -> (error out=w795:errorcluster)  [unwired: 1 in, 2 out]
          }
          frame "GetConfig_" {
            # "solution:\n\n1 call vi ref, vi send out typed command. => possible, idea, time consuming \n\n2 make this frame specific, bad. \n\n3 user event call and wait, then send typed command.  possible, fast?"
            n246 = Variant To Data(type=refnum<queue> refnum ("queue out"), Variant=w811) -> (data=w810:refnum<queue>, error out=w809:errorcluster)  [unwired: 1 in]
            n247 = case shown="No Error" w809 {
              selector: w809 -> [_ w820]
              tunnel: w810 -> [w819 _]
              tunnel: w808 -> [w816 _]
              tunnel: [w818 w820] -> w807
              tunnel: w806 -> [w817 _]
              frame No Error {
                # "short term solution, need refine\nget real result from device"
                n248 = Enqueue Element(queue=w819, element=w816, error in (no error)=w817) -> (error out=w818:errorcluster)  [unwired: 1 in, 2 out]
              }
              frame Error {
              }
            }
          }
          frame "==ModeSetup==" {
            # "Invalid Frame"
            n249 = xnode "Error Ring"() -> ("error out"=w823:errorcluster)
          }
          frame "SetSignalBuffer_" {
            n250 = Variant To Data(type=w841, Variant=w843) -> (data=w840:refnum<queue>, error out=w837:errorcluster)  [unwired: 1 in]
            n251 = Select(t=w841, s=w837, f=w840) -> (s? t:f=w842:refnum<queue>)
            n252 = xnode "Error Ring"() -> ("error out"=w836:errorcluster)
            n253 = Select(t=w836, s=w837, f=w838) -> (s? t:f=w839:errorcluster)
          }
          frame "SetMode_" {
            n254 = Unbundle By Name(w861) -> ("Mode(Gage)"=w858:T6)
            n255 = Variant To Data(error in=w855, type=w858, Variant=w860) -> (data=w857:T6, error out=w856:errorcluster)
            n256 = Select(t=w858, s=w856, f=w857) -> (s? t:f=w859:T6)
            n257 = Bundle By Name(cluster=w861, "Mode(Gage)"=w859) -> (w862:T1)
            n258 = disable-structure shown="Disabled" {
              frame Disabled {
                n259 = case shown="True" {
                  selector: _ -> [_ _]
                  frame False {
                  }
                  frame True {
                    # "for multirecord  and hwaverage"
                    n260 = call <instrlib>:"CsTool-ConfigureTimeStamp.vi"() -> ()  [unwired: 3 in, 1 out]
                  }
                }
              }
              frame Enabled {
              }
            }
          }
          frame "SetSecondaryDataRef._" {
            n261 = Variant To Data(type=T9 {"SecondaryDataVIRef."=refnum, "Option"=0} ("SecondaryDataParams."), Variant=w871) -> (data=w869:T9, error out=w870:errorcluster)  [unwired: 1 in]
            n262 = case shown="No Error" w870 {
              tunnel: w868 -> [w893 w897]
              tunnel: [w892 w897] -> w873
              tunnel: w869 -> [w888 _]
              tunnel: w868 -> [w885 _]
              tunnel: [w880 w896] -> w867
              frame No Error {
                n263 = Unbundle By Name(w885) -> ("SecondaryDataVIRef"=w883:refnum<vi>)
                n264 = Unbundle By Name(w888) -> ("SecondaryDataVIRef."=w887:refnum<vi>, "Option"=w886:i32)
                n265 = Not A Number/Path/Refnum?(number/path/refnum=w883) -> (NaN/Path/Refnum?=w884:bool)
                n266 = case shown="False" w884 {
                  tunnel: w883 -> [w895 _]
                  tunnel: [w894 _] -> w882
                  frame False {
                    n267 = Close Reference(reference=w895) -> (error out=w894:errorcluster)  [unwired: 1 in]
                  }
                  frame True {
                  }
                }
                n268 = property class="VI Interface Type 0"(reference=w887, error in=w882) -> (reference out=w890:refnum<vi>, error out=w881:errorcluster, "Path"=w891:path)
                n269 = Open VI Reference(type specifier VI Refnum (for type only)=w890, vi path=w891, error in (no error)=w881) -> (vi reference=w889:refnum<vi>, error out=w880:errorcluster)  [unwired: 3 in]
                n270 = Bundle By Name(cluster=w893, "SecondaryDataVIRef"=w889, "Option(SecondaryDataVI)"=w886) -> (w892:T1)
              }
              frame Error {
                n271 = xnode "Error Ring"() -> ("error out"=w896:errorcluster)
              }
            }
          }
        }
      }
      frame Error {
        n272 = xnode "Error Ring"() -> ("error out"=w905:errorcluster)
      }
    }
    n273 = call <vilib>:"Clear Errors.vi"("error in (no error)"=w50) -> ("error out"=w49:errorcluster)  [unwired: 6 in]
    "Core#" <- w51
  }
  "error out" <- w15
  n274 = while {
    tunnel: w22 -> [w924]
    tunnel: w5 -> [w923]
    tunnel: w20 -> [w921]
    tunnel: w10 -> [w920]
    tunnel: [w919] -> w8
    tunnel: [w918] -> _
    tunnel: [w917] -> _
    stop <- w917 stop-if-true
    w922 = 50  # Should not be -1, or do not quit as subVI
    n275 = event shown="[0] Timeout" {
      selector: _ -> [_ _ _ _ _ _ _ _ _ _ _ _ _ _ _ _]
      dyn-events: _ -> [_ _ _ _ _ _ _ _ _ _ _ _ _ _ _ _]
      timeout: w922 -> [_ _ _ _ _ _ _ _ _ _ _ _ _ _ _ _]
      tunnel: w924 -> [w934 w950 w954 w958 w963 w965 w973 w977 w979 w981 w983 w985 w987 w989 w991 w993]
      tunnel: w923 -> [_ _ _ _ w960 _ _ _ _ _ _ _ _ _ _ _]
      tunnel: w921 -> [w933 _ _ _ _ _ _ _ _ _ _ _ _ _ _ _]
      tunnel: [_ _ _ _ _ _ TRUE _ _ _ _ _ _ _ _ _] -> w918
      tunnel: [w932 _ _ _ _ _ errorcluster {"status"=FALSE, "code"=0, "source"=""} ("error constant") _ _ _ _ _ _ _ _ _] -> w919
      event Timeout {
        w925 = 100 ("timeout in ms (-1)")
        n276 = event-data() -> ()  [unwired: 1 in, 1 out]
        n277 = Bundle By Name(cluster=T7 {"DWF States"=enum."GetStat_", "Variant"=variant} ("element"), "Variant"=w933) -> (w930:T7)
        n278 = Enqueue Element At Opposite End "To get LiveStat,\nIt has to be opposite end"(queue=w934, element=w930) -> (error out=w929:errorcluster)  [unwired: 2 in, 2 out]
        n279 = Dequeue Element(queue=w933, timeout in ms (-1)=w925, error in (no error)=w929) -> (element=w928:T1, timed out?=w926:bool, error out=w932:errorcluster)  [unwired: 1 out]
        n280 = case shown="False" w926 {
          tunnel: w928 -> [w943 w946]
          tunnel: [w942 w945] -> w927
          tunnel: w925 -> [w938 _]
          frame False {
            n281 = Unbundle By Name(w943) -> ("TrigCount"=w941:i32)
            n282 = feedback-in #1(w941) -> ()
            n283 = feedback #1(0 ("TrigCount")) -> (w940:i32)
            n284 = Subtract(x=w941, y=w940) -> (x-y=w939:i32)
            n285 = Compound Arithmetic op=MULTIPLY(w939, invert w938, 1000.0 ("value")) -> (w936:dbl)
            n286 = Bundle By Name(cluster=w943, "TrigRate(Hz)"=w936) -> (w942:T1)
          }
          frame True {
            n287 = Bundle By Name(cluster=w946, "Model"="timeout !") -> (w945:T1)
          }
        }
        "LiveStat" <- w927
      }
      event Value Change {
        n288 = event-data() -> ("NewVal"=w947:T11)  [unwired: 1 in]
        n289 = Bundle By Name(cluster=T7 {"DWF States"=enum."SetAcquisition_", "Variant"=variant} ("element"), "Variant"=w947) -> (w948:T7)
        n290 = Enqueue Element(queue=w950, element=w948) -> ()  [unwired: 2 in, 3 out]
      }
      event Value Change {
        n291 = event-data() -> ("NewVal"=w951:T13)  [unwired: 1 in]
        n292 = Bundle By Name(cluster=T7 {"DWF States"=enum."SetChannels_", "Variant"=variant} ("element"), "Variant"=w951) -> (w952:T7)
        n293 = Enqueue Element(queue=w954, element=w952) -> ()  [unwired: 2 in, 3 out]
      }
      event Value Change {
        n294 = event-data() -> ("NewVal"=w955:T15)  [unwired: 1 in]
        n295 = Bundle By Name(cluster=T7 {"DWF States"=enum."SetTrigger_", "Variant"=variant} ("element"), "Variant"=w955) -> (w956:T7)
        n296 = Enqueue Element(queue=w958, element=w956) -> ()  [unwired: 2 in, 3 out]
      }
      event "ConfigAll": Value Change {
        n297 = event-data() -> ()  [unwired: 1 in, 1 out]
        n298 = property class="Clust (strict)"(reference=w960) -> ("Value"=w959:T3)  [unwired: 1 in, 2 out]
        n299 = Bundle By Name(cluster=T7 {"DWF States"=enum."SetAll_AcquChTrig_", "Variant"=variant} ("element"), "Variant"=w959) -> (w961:T7)
        n300 = Enqueue Element(queue=w963, element=w961) -> ()  [unwired: 2 in, 3 out]
      }
      event "Get_ConfigAll": Value Change {
        n301 = event-data() -> ()  [unwired: 1 in, 1 out]
        n302 = for {
          tunnel: w965 -> [w969]
          shift-right: [w968] -> _
          shift-left: _ -> [w967]
          tunnel: T7[] [{"DWF States"=enum."GetAcquisition", "Variant"=variant}, {"DWF States"=enum."GetChannels", "Variant"=variant}, {"DWF States"=enum."GetTrigger", "Variant"=variant}] -> [w966] mode=indexing
          n303 = Enqueue Element(queue=w969, element=w966, error in (no error)=w967) -> (error out=w968:errorcluster)  [unwired: 1 in, 2 out]
        }
      }
      event "Quit": Value Change {
        n304 = event-data() -> ()  [unwired: 1 in, 1 out]
        n305 = Enqueue Element(queue=w973, element=T7 {"DWF States"=enum."Quit", "Variant"=variant}) -> ()  [unwired: 2 in, 3 out]
      }
      event Value Change {
        n306 = event-data() -> ("NewVal"=w974:T6)  [unwired: 1 in]
        n307 = Bundle By Name(cluster=T7 {"DWF States"=enum."SetMode_", "Variant"=variant} ("element"), "Variant"=w974) -> (w975:T7)
        n308 = Enqueue Element(queue=w977, element=w975) -> ()  [unwired: 2 in, 3 out]
      }
      event "fConfig": Value Change {
        n309 = event-data() -> ()  [unwired: 1 in, 1 out]
        n310 = Enqueue Element(queue=w979, element=T7 {"DWF States"=enum."fConfigurate", "Variant"=variant}) -> ()  [unwired: 2 in, 3 out]
      }
      event "Start": Value Change {
        n311 = event-data() -> ()  [unwired: 1 in, 1 out]
        n312 = Enqueue Element(queue=w981, element=T7 {"DWF States"=enum."fStart", "Variant"=variant}) -> ()  [unwired: 2 in, 3 out]
      }
      event "Reset": Value Change {
        n313 = event-data() -> ()  [unwired: 1 in, 1 out]
        n314 = Enqueue Element(queue=w983, element=T7 {"DWF States"=enum."Quit", "Variant"=variant}) -> ()  [unwired: 2 in, 3 out]
      }
      event "CloseAll": Value Change {
        n315 = event-data() -> ()  [unwired: 1 in, 1 out]
        n316 = Enqueue Element(queue=w985, element=T7 {"DWF States"=enum."CloseAll", "Variant"=variant}) -> ()  [unwired: 2 in, 3 out]
      }
      event "Close": Value Change {
        n317 = event-data() -> ()  [unwired: 1 in, 1 out]
        n318 = Enqueue Element(queue=w987, element=T7 {"DWF States"=enum."Close", "Variant"=variant}) -> ()  [unwired: 2 in, 3 out]
      }
      event "Open": Value Change {
        n319 = event-data() -> ()  [unwired: 1 in, 1 out]
        n320 = Enqueue Element(queue=w989, element=T7 {"DWF States"=enum."Open", "Variant"=variant}) -> ()  [unwired: 2 in, 3 out]
      }
      event "Enumerate": Value Change {
        n321 = event-data() -> ()  [unwired: 1 in, 1 out]
        n322 = Enqueue Element(queue=w991, element=T7 {"DWF States"=enum."Enumerate", "Variant"=variant}) -> ()  [unwired: 2 in, 3 out]
      }
      event "StartAll": Value Change {
        n323 = event-data() -> ()  [unwired: 1 in, 1 out]
        n324 = property on="Gage_Config" class="Clust (strict)"() -> ("Value"=w992:T3)  [unwired: 2 in, 2 out]
        n325 = Bundle By Name(cluster=T7 {"DWF States"=enum."SetAll_AcquChTrig_", "Variant"=variant} ("element"), "Variant"=w992) -> (w997:T7)
        n326 = Build Array(T7 {"DWF States"=enum."Enumerate", "Variant"=variant} ("element"), T7 {"DWF States"=enum."Open", "Variant"=variant} ("element"), w997, T7 {"DWF States"=enum."fConfigurate", "Variant"=variant} ("element"), T7 {"DWF States"=enum."fStart", "Variant"=variant} ("element")) -> (w1000:T7[])
        n327 = for {
          shift-right: [w1004] -> _
          shift-left: w993 -> [w1005]
          tunnel: w1000 -> [w1003] mode=indexing
          shift-right: [w1002] -> _
          shift-left: _ -> [w1001]
          n328 = Enqueue Element(queue=w1005, element=w1003, error in (no error)=w1001) -> (queue out=w1004:refnum<queue>, error out=w1002:errorcluster)  [unwired: 1 in, 1 out]
        }
      }
    }
    n329 = Or(x=w918, y=w920) -> (x .or. y?=w917:bool)
  }
  n330 = Release Queue(queue=w17, error in (no error)=w15) -> (error out=w21:errorcluster)  [unwired: 1 in, 2 out]
  n331 = Release Queue(queue=w22, error in (no error)=w21) -> (error out=w19:errorcluster)  [unwired: 1 in, 2 out]
  n332 = Merge Errors(w8, w19) -> (w9:errorcluster)
  n333 = Release Queue(queue=w20, error in (no error)=w9) -> (error out=w14:errorcluster)  [unwired: 1 in, 2 out]
  n334 = call <vilib>:"General Error Handler.vi"("type of dialog (OK msg:1)"=w13, "error in (no error)"=w14, "[exception action] (none:0)"=w12, "[exception code]"=w11) -> ()  [unwired: 7 in, 5 out]
